vi "Test Sync with Queues.vi"() -> ()   [LabVIEW 2019, in "DAQmx.lvclass"]
uses:
  DAQmx.lvclass
  typedefs/DAQ.Config.Timing.Sampling--Cluster.ctl
  typedefs/DAQ.Config.AO--Cluster--Array.ctl
  typedefs/DAQ.Config.AO--Cluster.ctl
  typedefs/DAQ.Config.AO.Range--enum.ctl
  typedefs/DAQ.Config.Device Type--enum.ctl
  typedefs/DAQ.Config.AI--Cluster--Array.ctl
  typedefs/DAQ.Config.AI--Cluster.ctl
  typedefs/DAQ.Config.AI.Coupling--enum.ctl
  typedefs/DAQ.Config.AI.Range--enum.ctl
  typedefs/DAQ.Configuration--Cluster.ctl
  typedefs/DAQ.Config.Timing--Cluster.ctl
  DAQmx.lvclass/DAQmx.ctl
panel:
  in  "AI":T1 {"input terminal configuration" items=[""=-1, "Differential"=10106, "Pseudodifferential"=12529]; "Coupling" items=[""=0, "AC"=10045, "DC"=10050, "GND"=10066]}
  in  "AO":T6 {"output terminal configuration" items=[""=-1, "Differential"=10106, "Pseudodifferential"=12529]}
  in  "Sampling":T9={"Fs"=52000.0, "#s"=5000} {"Fs" format="%#_13g"}
  out "Waveform Chart":i32(graph)
  out "Generator create":i32
  out "Generator 'timeout'":i32
  out "DAQ 'timeout'":i32
  out "Generator":i32
  out "DAQ":i32
  out "Waveform Graph":waveform(dbl)[](graph)
  in  "stop":bool
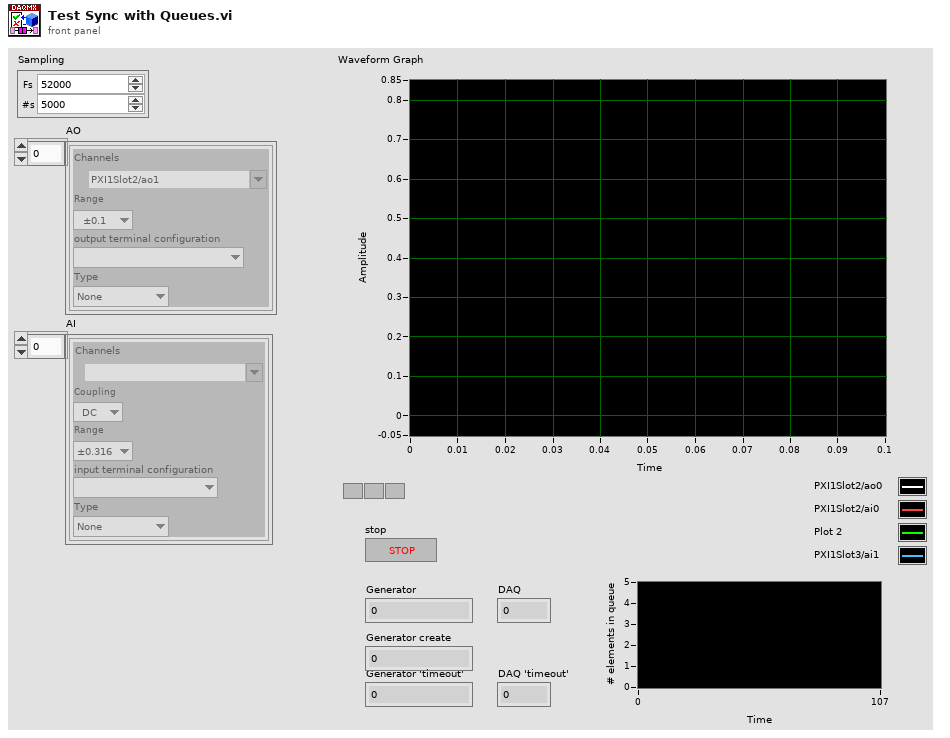
[diagram p1: front panel]
types:
  T1 = typedef "DAQmx.lvclass/DAQ.Config.AI--Cluster--Array.ctl" = T2[]
  T2 = typedef "DAQmx.lvclass/DAQ.Config.AI--Cluster.ctl" = cluster{"Channels":tag, "Coupling":T3, "Range":T4, "input terminal configuration":i32, "Type":T5}
  T3 = typedef "DAQmx.lvclass/DAQ.Config.AI.Coupling--enum.ctl" = u16
  T4 = typedef "DAQmx.lvclass/DAQ.Config.AI.Range--enum.ctl" = enum16{"±0.316", "±1.00", "±3.16", "±10.0", "±31.6", "±42.4", ""}
  T5 = typedef "DAQmx.lvclass/DAQ.Config.Device Type--enum.ctl" = enum16{"None", "USB-4431", "PXI-446x"}
  T6 = typedef "DAQmx.lvclass/DAQ.Config.AO--Cluster--Array.ctl" = T7[]
  T7 = typedef "DAQmx.lvclass/DAQ.Config.AO--Cluster.ctl" = cluster{"Channels":tag, "Range":T8, "output terminal configuration":i32, "Type":T5}
  T8 = typedef "DAQmx.lvclass/DAQ.Config.AO.Range--enum.ctl" = enum16{"±0.1", "±1.0", "±3.5", "±10.0", ""}
  T9 = typedef "DAQmx.lvclass/DAQ.Config.Timing.Sampling--Cluster.ctl" = cluster{"Fs":dbl, "#s":i32}
  T10 = typedef "DAQmx.lvclass/DAQ.Configuration--Cluster.ctl" = cluster{"Timing":T11, "AO":T6, "AI":T1}
  T11 = typedef "DAQmx.lvclass/DAQ.Config.Timing--Cluster.ctl" = cluster{"Sampling":T9, "Fs_Out":dbl}
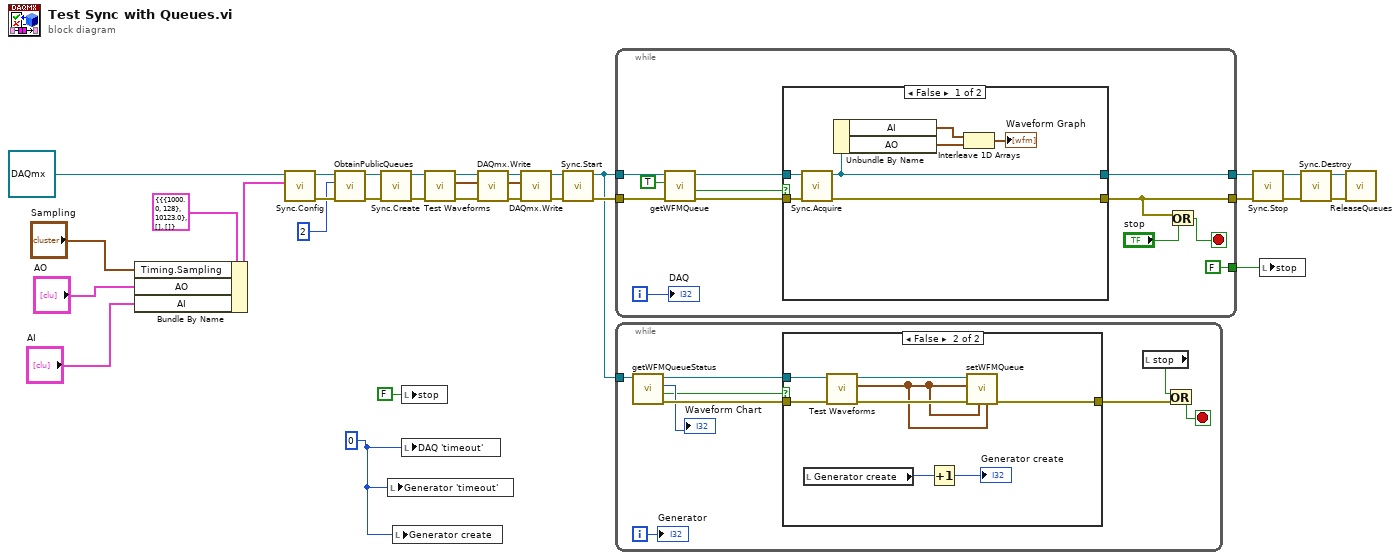
[diagram p0: block diagram]
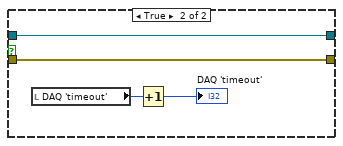
[diagram p2: hidden frame]
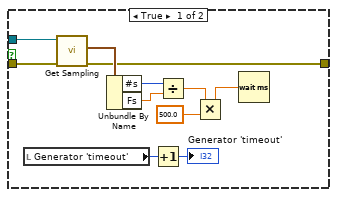
[diagram p3: hidden frame]
diagram:
  w28 = 0 ("consumer 2")
  n1 = Bundle By Name(cluster=T10 {"Timing"={"Sampling"={"Fs"=1000.0, "#s"=128}, "Fs_Out"=10123.0}, "AO"=[], "AI"=[]} ("Configuration"), "Timing.Sampling"="Sampling", "AO"="AO", "AI"="AI") -> (w12:T10)
  n2 = call "Sync.Config.vi"("Configuration"=w12, "DAQmx in"=refnum<class "DAQmx.lvclass"> refnum) -> ("error out"=w14:errorcluster, "DAQmx out"=w15:refnum<class "DAQmx.lvclass">)  [unwired: 8 in]
  n3 = call "ObtainPublicQueues.vi"("error in (no error)"=w14, "Min Queue Buffer"=2, "DAQmx"=w15) -> ("error out"=w21:errorcluster, "DAQmx out"=w22:refnum<class "DAQmx.lvclass">)  [unwired: 7 in]
  n4 = call "Sync.Create.vi"("error in"=w21, "DAQmx in"=w22) -> ("error out"=w24:errorcluster, "DAQmx out"=w25:refnum<class "DAQmx.lvclass">)  [unwired: 8 in]
  n5 = local write "Generator 'timeout'"(w28) -> ()
  n6 = local write "Generator create"(w28) -> ()
  n7 = local write "stop"(FALSE ("stop")) -> ()
  n8 = local write "DAQ 'timeout'"(w28) -> ()
  n9 = call "Test Waveforms.vi"("error in (no error)"=w24, "DAQmx in"=w25) -> ("error out"=w3:errorcluster, "Waveforms"=w4:waveform(dbl)[], "DAQmx out"=w7:refnum<class "DAQmx.lvclass">)  [unwired: 7 in]
  n10 = call "DAQmx.Write.vi"("error in (no error)"=w3, "AOwfm"=w4, "DAQmx in"=w7) -> ("error out"=w5:errorcluster, "DAQmx out"=w6:refnum<class "DAQmx.lvclass">)  [unwired: 6 in, 1 out]
  n11 = call "DAQmx.Write.vi"("error in (no error)"=w5, "AOwfm"=w4, "DAQmx in"=w6) -> ("error out"=w2:errorcluster, "DAQmx out"=w1:refnum<class "DAQmx.lvclass">)  [unwired: 6 in, 1 out]
  n12 = call "Sync.Start.vi"("error in"=w2, "DAQmx in"=w1) -> ("error out"=w26:errorcluster, "DAQmx out"=w23:refnum<class "DAQmx.lvclass">)  [unwired: 8 in]
  n13 = while {
    tunnel: w23 -> [w36]
    tunnel: [w43] -> w31
    tunnel: [w39] -> w30
    tunnel: w26 -> [w33]
    tunnel: [FALSE ("stop")] -> w27
    i -> [w40]
    stop <- w41 stop-if-true
    n14 = call "getWFMQueue.vi"("error in (no error)"=w33, "wait for min buffer?"=TRUE, "DAQmx in"=w36) -> ("error out"=w34:errorcluster, "timed out?"=w35:bool, "DAQmx out"=w37:refnum<class "DAQmx.lvclass">)  [unwired: 6 in]
    n15 = case shown="False" w35 {
      tunnel: [w44 w54] -> w43
      tunnel: [w49 w53] -> w39
      tunnel: w37 -> [w48 w54]
      tunnel: w34 -> [w47 w53]
      frame False {
        n16 = call "Sync.Acquire.vi"("error in (no error)"=w47, "DAQmx in"=w48) -> ("error out"=w49:errorcluster, "DAQmx out"=w44:refnum<class "DAQmx.lvclass">)  [unwired: 8 in]
        n17 = Unbundle By Name(w44) -> ("AI"=w46:waveform(dbl)[], "AO"=w45:waveform(dbl)[])
        n18 = Interleave 1D Arrays(w46, w45) -> (→"Waveform Graph":waveform(dbl)[])
      }
      frame True {
        n19 = local read "DAQ 'timeout'"() -> (w52:i32)
        n20 = Increment(x=w52) -> (x+1=→"DAQ 'timeout'":i32)
      }
    }
    n21 = Or(x=w39, y="stop") -> (x .or. y?=w41:bool)
    "DAQ" <- w40
  }
  n22 = while {
    tunnel: w23 -> [w59]
    i -> [w63]
    stop <- w61 stop-if-true
    n23 = call "getWFMQueueStatus.vi"("DAQmx in"=w59) -> ("error out"=w58:errorcluster, "Min AO Queue Filled"=w55:bool, "AO queue #"=→"Waveform Chart":i32, "DAQmx out"=w60:refnum<class "DAQmx.lvclass">)  [unwired: 7 in]
    n24 = case shown="False" w55 {
      tunnel: w60 -> [w67 w80]
      tunnel: w58 -> [w66 w78]
      tunnel: [w64 w76] -> w57
      frame True {
        n25 = local read "Generator 'timeout'"() -> (w74:i32)
        n26 = call "Get Sampling.vi"("error in (no error)"=w66, "DAQmx in"=w67) -> ("error out"=w64:errorcluster, "Sampling info"=w65:T9)  [unwired: 7 in, 1 out]
        n27 = Unbundle By Name(w65) -> ("#s"=w72:i32, "Fs"=w71:dbl)
        n28 = Increment(x=w74) -> (x+1=→"Generator 'timeout'":i32)
        n29 = Divide(x=w72, y=w71) -> (x/y=w69:dbl)
        n30 = Multiply(x=w69, y=500.0) -> (x*y=w68:dbl)
        n31 = Wait (ms)(milliseconds to wait=w68) -> ()  [unwired: 1 out]
      }
      frame False {
        n32 = local read "Generator create"() -> (w81:i32)
        n33 = call "Test Waveforms.vi"("error in (no error)"=w78, "DAQmx in"=w80) -> ("error out"=w77:errorcluster, "Waveforms"=w75:waveform(dbl)[], "DAQmx out"=w79:refnum<class "DAQmx.lvclass">)  [unwired: 7 in]
        n34 = Increment(x=w81) -> (x+1=→"Generator create":i32)
        n35 = call "setWFMQueue.vi"("REF_Y"=w75, "REF_X"=w75, "error in (no error)"=w77, "AO"=w75, "DAQmx in"=w79) -> ("error out"=w76:errorcluster)  [unwired: 5 in, 1 out]
      }
    }
    n36 = local read "stop"() -> (w62:bool)
    n37 = Or(x=w62, y=w57) -> (x .or. y?=w61:bool)
    "Generator" <- w63
  }
  n38 = call "Sync.Stop.vi"("error in (no error)"=w30, "DAQmx in"=w31) -> ("error out"=w17:errorcluster, "DAQmx out"=w18:refnum<class "DAQmx.lvclass">)  [unwired: 8 in]
  n39 = local write "stop"(w27) -> ()
  n40 = call "Sync.Destroy.vi"("error in (no error)"=w17, "DAQmx in"=w18) -> ("error out"=w19:errorcluster, "DAQmx out"=w20:refnum<class "DAQmx.lvclass">)  [unwired: 8 in]
  n41 = call "ReleaseQueues.vi"("error in (no error)"=w19, "DAQmx"=w20) -> ()  [unwired: 8 in, 2 out]
